vi "REPORT_GEAR_get_operations_and_results.vi"(6 "executed_SQL_statement_in":string, 8 "error_in":errorcluster, 11 "SQL_result":variant) -> (0 "error_out":errorcluster, 4 "executed_SQL_statement_out":string)   [LabVIEW 2019]
uses:
  FGV/REPORTS_records_display/FGV_REPORTS_records_display.ctl
  FGV/SQL_connection/FGV_CLIENT_SQL_connection.ctl
  _misc/AULocalize/SubVIs/Get Localized Phrase Compact Interface 0D.vi
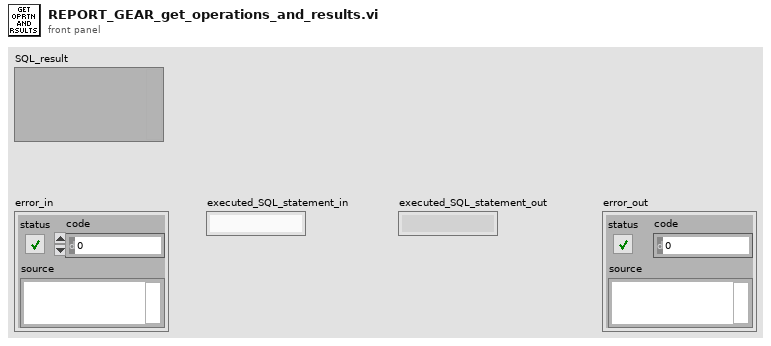
[diagram p1: front panel]
types:
  T1 = typedef "FGV_REPORTS_records_display.ctl" = enum16{"initialize", "GEAR_set_serial", "GEAR_set_header", "GEAR_set_operations", "GEAR_set_results", "GEAR_set_batches", "GEAR_get_serial", "GEAR_get_operation_IDs", "GEAR_toggle_results", "GEAR_show_all_results", "GEAR_hide_all_results", "GEAR_display", "GEAR_filter", "GEAR_restore", "GEAR_clear", "GEAR_get_all_info", "DATES_set_dates", "DATES_set_gears", "DATES_display", "DATES_filter", "DATES_first_page", "DATES_previous_page", "DATES_next_page", "DATES_last_page", "DATES_restore", "DATES_clear", "DATES_get_all_info", "PBATCH_set_batch_no", "PBATCH_set_gears", "PBATCH_display", "PBATCH_filter", "PBATCH_first_page", "PBATCH_previous_page", "PBATCH_next_page", "PBATCH_last_page", "PBATCH_restore", "PBATCH_clear", "PBATCH_get_all_info", "OPRTN_set_OP", "OPRTN_set_dates", "OPRTN_set_gears", "OPRTN_set_hidden_columns", "OPRTN_display", "OPRTN_filter", "OPRTN_filter_no_page_reset", "OPRTN_first_page", "OPRTN_previous_page", "OPRTN_next_page", "OPRTN_last_page", "OPRTN_restore", "OPRTN_clear", "OPRTN_get_all_info", "CFG_set_type", "CFG_set_dates", "CFG_set_records", "CFG_display", "CFG_filter", "CFG_first_page", "CFG_previous_page", "CFG_next_page", "CFG_last_page", "CFG_restore", "CFG_clear", "CFG_get_all_info", "AUDIT_set_dates", "AUDIT_set_records", "AUDIT_display", "AUDIT_filter", "AUDIT_first_page", "AUDIT_previous_page", "AUDIT_next_page", "AUDIT_last_page", "AUDIT_restore", "AUDIT_clear", "AUDIT_get_all_info", "OKNOK_set_dates", "OKNOK_set_records", "OKNOK_display", "OKNOK_restore", "OKNOK_clear", "OKNOK_get_all_info", "REWORKS_set_dates", "REWORKS_set_from_to", "REWORKS_set_records", "REWORKS_display", "REWORKS_filter", "REWORKS_first_page", "REWORKS_previous_page", "REWORKS_next_page", "REWORKS_last_page", "REWORKS_restore", "REWORKS_clear", "REWORKS_get_all_info", "PACE_set_dates", "PACE_set_limits", "PACE_set_records", "PACE_display", "PACE_restore", "PACE_clear", "PACE_get_all_info", "CBATCH_set_code", "CBATCH_set_records", "CBATCH_display", "CBATCH_filter", "CBATCH_first_page", "CBATCH_previous_page", "CBATCH_next_page", "CBATCH_last_page", "CBATCH_restore", "CBATCH_clear", "CBATCH_get_all_info", "CMPNT_set_serial", "CMPNT_set_records", "CMPNT_display", "CMPNT_first_page", "CMPNT_previous_page", "CMPNT_next_page", "CMPNT_last_page", "CMPNT_restore", "CMPNT_clear", "CMPNT_get_all_info", "clear"}
  T2 = typedef "FGV_CLIENT_SQL_connection.ctl" = enum16{"initialize", "connect", "read_tables", "read_columns", "SELECT", "INSERT", "UPDATE", "DELETE", "EXEC + headers", "EXEC", "TRANSACTION", "connection_active?", "disconnect"}
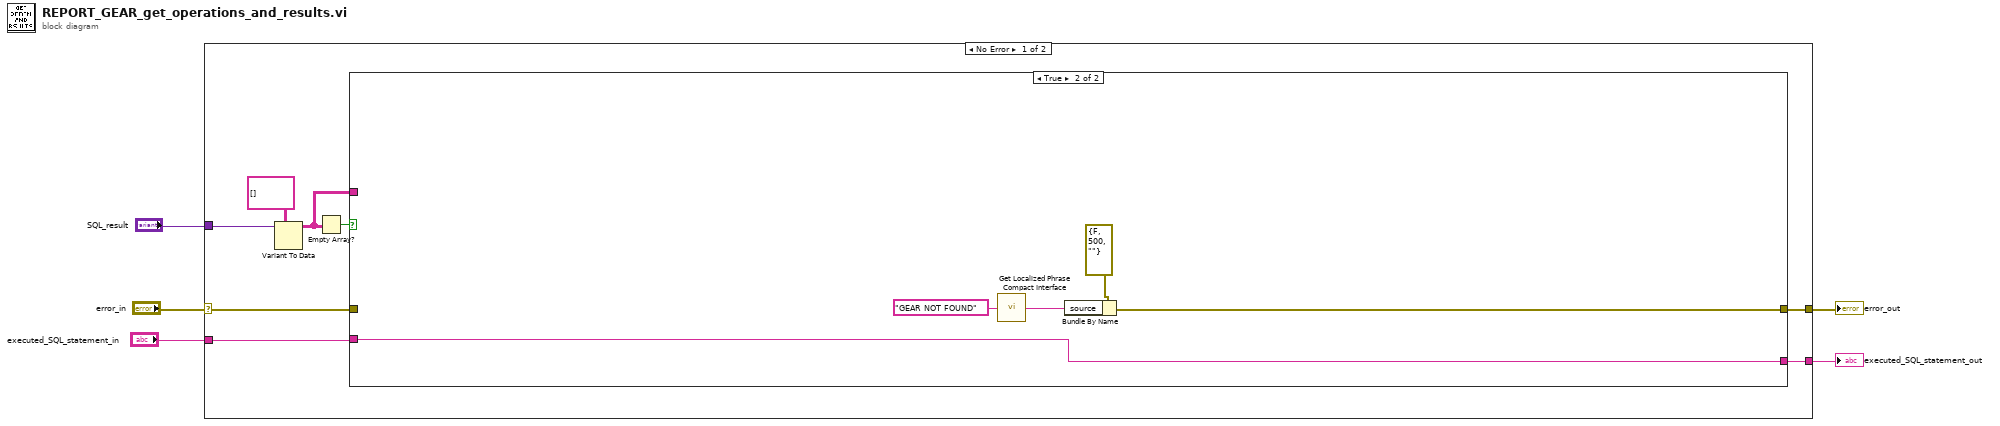
[diagram p0: block diagram]
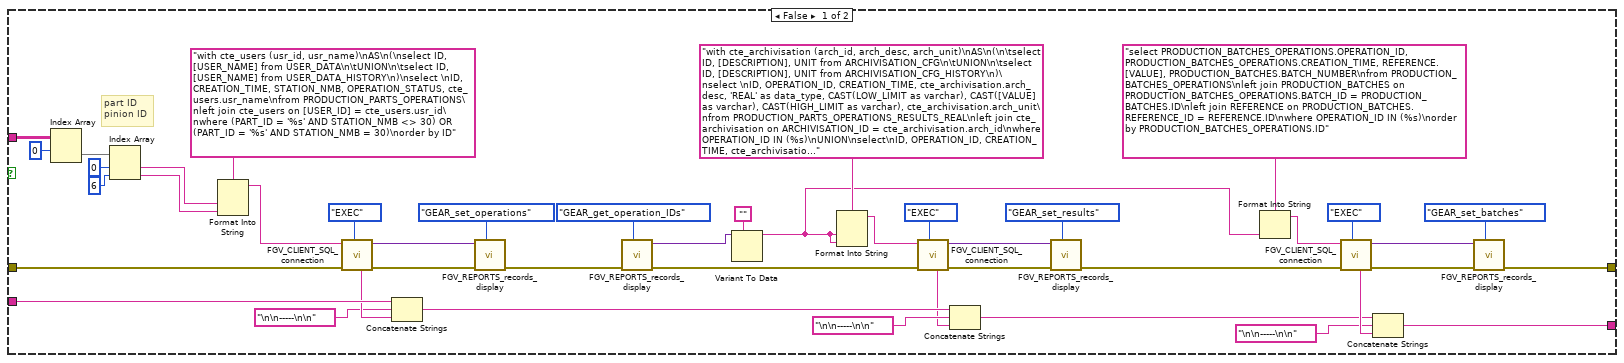
[diagram p2: hidden frame]
diagram:
  n1 = case shown="No Error" "error_in" {
    selector: "error_in" -> [w10 w64]
    tunnel: [w13 w63] -> w5
    tunnel: "executed_SQL_statement_in" -> [w12 w63]
    tunnel: [w11 w64] -> w3
    tunnel: "SQL_result" -> [w9 _]
    frame No Error {
      n2 = Variant To Data(type=string[][] [], Variant=w9) -> (data=w7:string[][])  [unwired: 1 in, 1 out]
      n3 = Empty Array?(array=w7) -> (empty?=w8:bool)
      n4 = case shown="True" w8 {
        tunnel: w10 -> [w57 _]
        tunnel: [w17 w58] -> w11
        tunnel: w12 -> [w43 w62]
        tunnel: [w15 w62] -> w13
        tunnel: w7 -> [w52 _]
        frame False {
          # "part ID\npinion ID"
          n5 = Index Array(array=w52, index (row)=0) -> (element=w50:string[])  [unwired: 1 in]
          n6 = Index Array(array=w50, index #1=0 ("index"), index #2=6 ("index")) -> (element #1=w45:string, element #2=w44:string)
          n7 = Format Into String(format string="with cte_users (usr_id, usr_name)\nAS\n(\nselect ID, [USER_NAME] from USER_DATA\n\tUNION\n\tselect ID, [USER_NAME] from USER_DATA_HISTORY\n)\nselect \nID, CREATION_TIME, STATION_NMB, OPERATION_STATUS, cte_users.usr_name\nfrom PRODUCTION_PARTS_OPERATIONS\nleft join cte_users on [USER_ID] = cte_users.usr_id\nwhere (PART_ID = '%s' AND STATION_NMB <> 30) OR (PART_ID = '%s' AND STATION_NMB = 30)\norder by ID", w45, w44) -> (resulting string=w47:string)  [unwired: 2 in, 1 out]
          n8 = call "FGV_CLIENT_SQL_connection.vi"("options"=FGV_CLIENT_SQL_connection."EXEC", "error_in"=w57, "SQL_statement"=w47) -> ("error_out"=w54:errorcluster, "SQL_result"=w53:variant, "executed_SQL_statement"=w42:string)  [unwired: 4 in, 2 out]
          n9 = Concatenate Strings(w43, "\n\n-----\n\n" ("string"), w42) -> (w35:string)
          n10 = call "FGV_REPORTS_records_display.vi"("options"=FGV_REPORTS_records_display."GEAR_set_operations", "error_in"=w54, "input"=w53) -> ("error_out"=w31:errorcluster)  [unwired: 7 in, 1 out]
          n11 = call "FGV_REPORTS_records_display.vi"("options"=FGV_REPORTS_records_display."GEAR_get_operation_IDs", "error_in"=w31) -> ("error_out"=w30:errorcluster, "output"=w28:variant)  [unwired: 8 in]
          n12 = Variant To Data(type="", Variant=w28) -> (data=w14:string)  [unwired: 1 in, 1 out]
          n13 = Format Into String(format string="with cte_archivisation (arch_id, arch_desc, arch_unit)\nAS\n(\n\tselect ID, [DESCRIPTION], UNIT from ARCHIVISATION_CFG\n\tUNION\n\tselect ID, [DESCRIPTION], UNIT from ARCHIVISATION_CFG_HISTORY\n)\nselect \nID, OPERATION_ID, CREATION_TIME, cte_archivisation.arch_desc, 'REAL' as data_type, CAST(LOW_LIMIT as varchar), CAST([VALUE] as varchar), CAST(HIGH_LIMIT as varchar), cte_archivisation.arch_unit\nfrom PRODUCTION_PARTS_OPERATIONS_RESULTS_REAL\nleft join cte_archivisation on ARCHIVISATION_ID = cte_archivisation.arch_id\nwhere OPERATION_ID IN (%s)\nUNION\nselect\nID, OPERATION_ID, CREATION_TIME, cte_archivisation.arch_desc, 'STRING' as data_type, '-', [VALUE], '-', cte_archivisation.arch_unit\nfrom PRODUCTION_PARTS_OPERATIONS_RESULTS_STRING\nleft join cte_archivisation on ARCHIVISATION_ID = cte_archivisation.arch_id\nwhere OPERATION_ID IN (%s)\norder by data_type, ID", w14, w14) -> (resulting string=w33:string)  [unwired: 2 in, 1 out]
          n14 = call "FGV_CLIENT_SQL_connection.vi"("options"=FGV_CLIENT_SQL_connection."EXEC", "error_in"=w30, "SQL_statement"=w33) -> ("error_out"=w38:errorcluster, "SQL_result"=w40:variant, "executed_SQL_statement"=w34:string)  [unwired: 4 in, 2 out]
          n15 = Concatenate Strings(w35, "\n\n-----\n\n" ("string"), w34) -> (w16:string)
          n16 = call "FGV_REPORTS_records_display.vi"("options"=FGV_REPORTS_records_display."GEAR_set_results", "error_in"=w38, "input"=w40) -> ("error_out"=w18:errorcluster)  [unwired: 7 in, 1 out]
          n17 = Format Into String(format string="select PRODUCTION_BATCHES_OPERATIONS.OPERATION_ID, PRODUCTION_BATCHES_OPERATIONS.CREATION_TIME, REFERENCE.[VALUE], PRODUCTION_BATCHES.BATCH_NUMBER\nfrom PRODUCTION_BATCHES_OPERATIONS\nleft join PRODUCTION_BATCHES on PRODUCTION_BATCHES_OPERATIONS.BATCH_ID = PRODUCTION_BATCHES.ID\nleft join REFERENCE on PRODUCTION_BATCHES.REFERENCE_ID = REFERENCE.ID\nwhere OPERATION_ID IN (%s)\norder by PRODUCTION_BATCHES_OPERATIONS.ID", w14) -> (resulting string=w25:string)  [unwired: 2 in, 1 out]
          n18 = call "FGV_CLIENT_SQL_connection.vi"("options"=FGV_CLIENT_SQL_connection."EXEC", "error_in"=w18, "SQL_statement"=w25) -> ("error_out"=w21:errorcluster, "SQL_result"=w19:variant, "executed_SQL_statement"=w24:string)  [unwired: 4 in, 2 out]
          n19 = Concatenate Strings(w16, "\n\n-----\n\n" ("string"), w24) -> (w15:string)
          n20 = call "FGV_REPORTS_records_display.vi"("options"=FGV_REPORTS_records_display."GEAR_set_batches", "error_in"=w21, "input"=w19) -> ("error_out"=w17:errorcluster)  [unwired: 7 in, 1 out]
        }
        frame True {
          n21 = call-poly "Get Localized Phrase Compact Interface.vi"("Key"="GEAR NOT FOUND" ("source")) -> ("Translated Phrase"=w59:string)
          n22 = Bundle By Name(cluster=errorcluster {"status"=FALSE, "code"=500, "source"=""} ("error IO"), "source"=w59) -> (w58:errorcluster)
        }
      }
    }
    frame Error {
    }
  }
  "executed_SQL_statement_out" <- w5
  "error_out" <- w3
